vi "DriveWaitForTime.vi"(2 "Parameter String":string, 3 "Reinit":bool) -> (0 "Error Out":errorcluster, 1 "Increment":bool)   [LabVIEW 2023]
doc: "This VI pauses the drive sequencer until the elapsed time has passed.\n\nParameters:\nParam1: time delay (ms) or if -1 from the dashboard (s)"
uses:
  SafeParser_Integer.vi
  GlobalDriverStationCommands.vi
  GlobalDriverStationData.vi
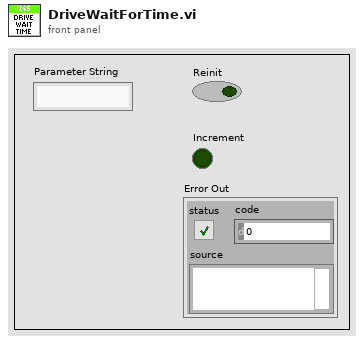
[diagram p1: front panel]
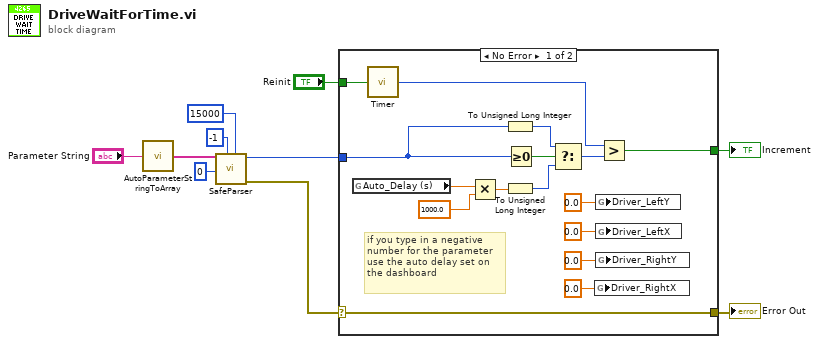
[diagram p0: block diagram]
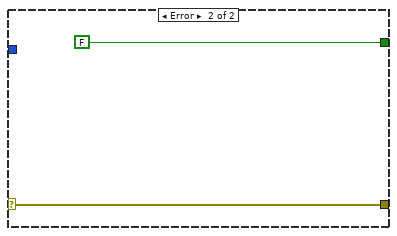
[diagram p2: hidden frame]
diagram:
  n1 = call "AutoParameterStringToArray.vi"("Parameter String"="Parameter String") -> ("Parsed Parameters"=w2:string[])
  n2 = call-poly "SafeParser.vi"("Maximum"=15000, "Minimum"=-1, "Array Index"=0 ("Parameter Index"), "String Array"=w2) -> ("Error Out"=w1:errorcluster, "Typecast  Value"=w6:i32)  [unwired: 6 in]
  n3 = case shown="No Error" w1 {
    selector: w1 -> [w19 w28]
    tunnel: [w22 FALSE] -> w10
    tunnel: "Reinit" -> [w21 _]
    tunnel: [w19 w28] -> w8
    tunnel: w6 -> [w18 _]
    frame No Error {
      # "if you type in a negative\nnumber for the parameter\nuse the auto delay set on \nthe dashboard"
      n4 = global read "GlobalDriverStationData.vi" "Auto_Delay (s)"() -> (w15:dbl)
      n5 = call "Timer.vi"("Reset Timer"=w21) -> ("Time (ms)"=w20:u32)
      n6 = Multiply(x=w15, y=1000.0) -> (x*y=w16:dbl)
      n7 = To Unsigned Long Integer(number=w18) -> (unsigned 32bit integer=w14:u32)
      n8 = To Unsigned Long Integer(number=w16) -> (unsigned 32bit integer=w17:u32)
      n9 = Greater Or Equal To 0?(x=w18) -> (x >= 0?=w13:bool)
      n10 = Select(t=w14, s=w13, f=w17) -> (s? t:f=w11:u32)
      n11 = global write "GlobalDriverStationCommands.vi" "Driver_RightX"(0.0 ("Driver_RightX")) -> ()
      n12 = global write "GlobalDriverStationCommands.vi" "Driver_LeftY"(0.0 ("Driver_LeftY")) -> ()
      n13 = global write "GlobalDriverStationCommands.vi" "Driver_LeftX"(0.0 ("Driver_RightX")) -> ()
      n14 = global write "GlobalDriverStationCommands.vi" "Driver_RightY"(0.0 ("Driver_RightX")) -> ()
      n15 = Greater?(x=w20, y=w11) -> (0:w22:bool)
    }
    frame Error {
    }
  }
  "Increment" <- w10
  "Error Out" <- w8
